vi "MainUI.vi"() -> ()   [LabVIEW 2017]
uses:
  QueueStates.ctl
  <vilib>/Instr/_visa.llb/VISA Configure Serial Port (Serial Instr).vi
panel:
  out "Phase Delta":dbl
  out "Gain":dbl
  out "Plot 1 PkPk":u16
  out "Plot 1 Min":u16
  out "Plot 1 Max":u16
  out "Plot 0 PkPk":u16
  in  "Sample Size":i32=1000
  out "Plot 0 Min":u16
  out "Plot 0 Max":u16
  out "Waveform Graph":u16[][](graph)
  out "String":string
  out "length":i32
  in  "Search Param":string="d"
  in  "STOP":bool
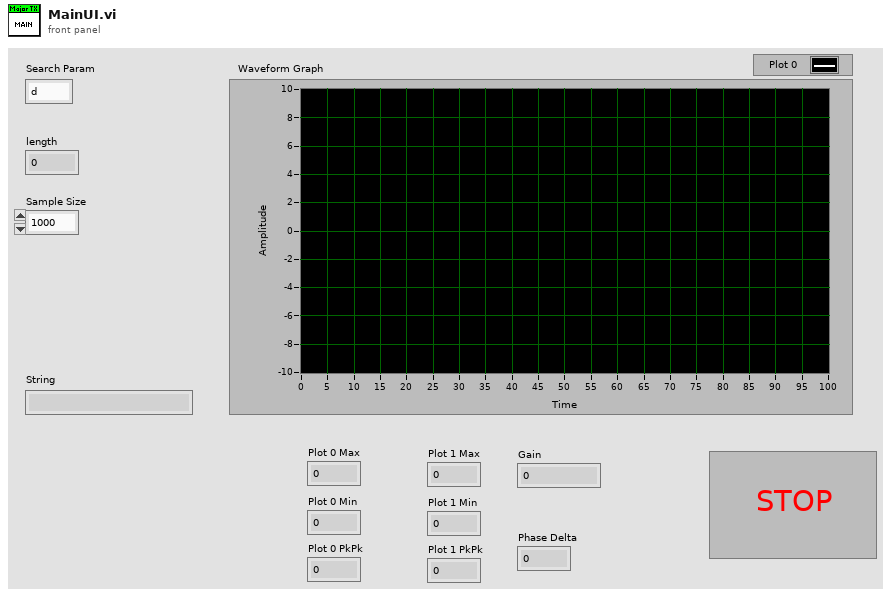
[diagram p1: front panel]
types:
  T1 = typedef "QueueStates.ctl" = enum16{"Init", "Exit", "Data", "CheckText", "Analyze"}
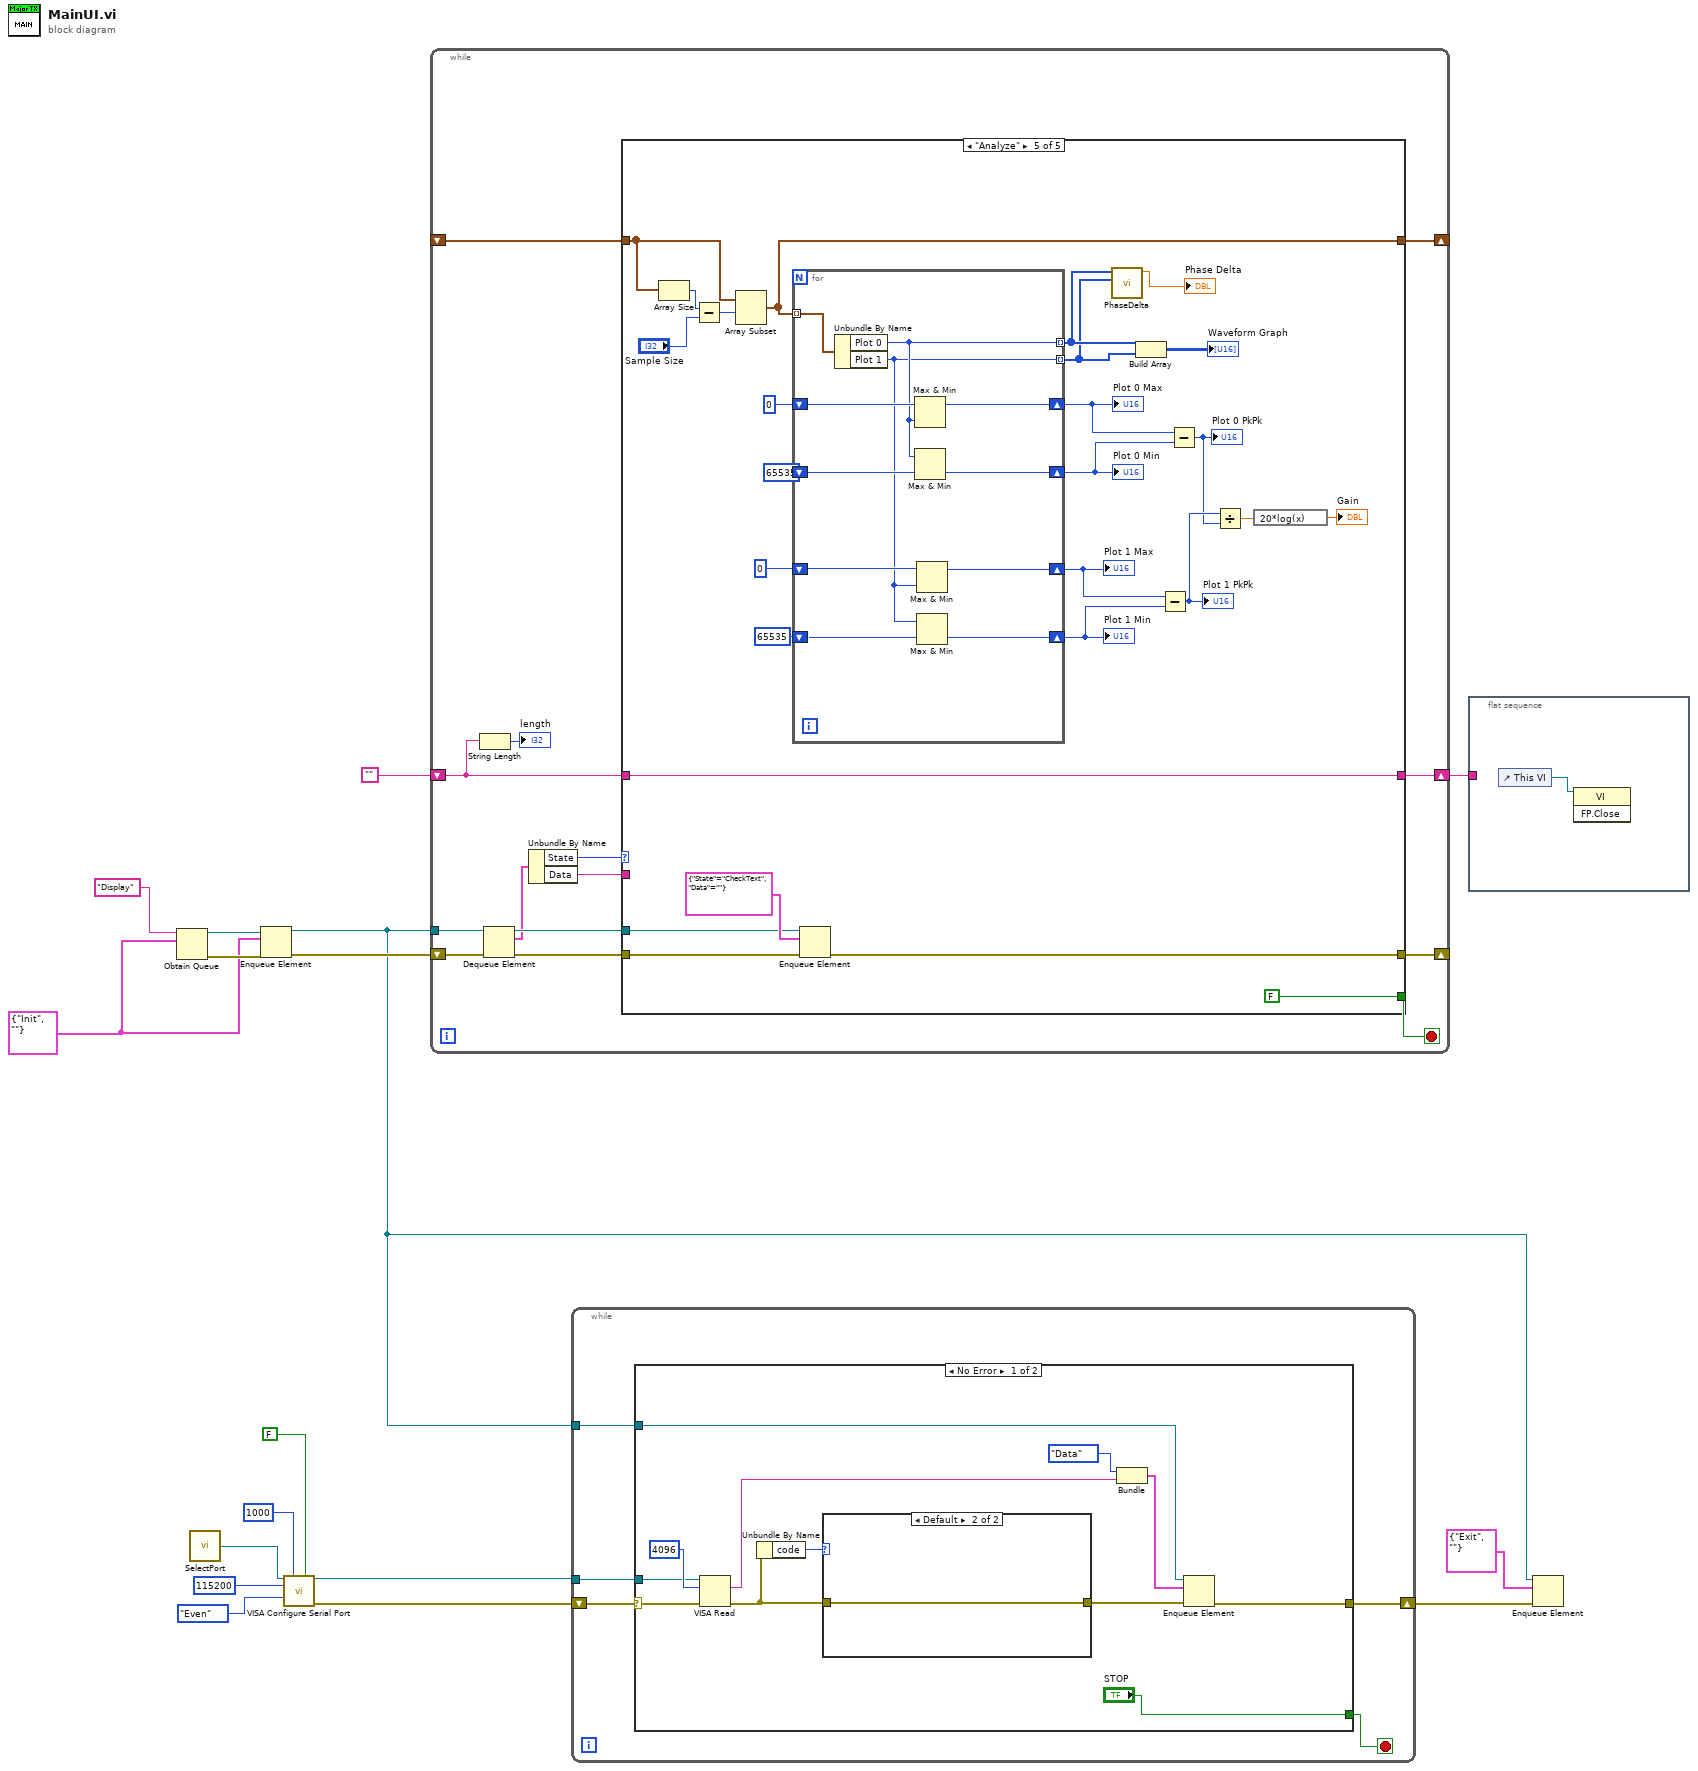
[diagram p0: block diagram]
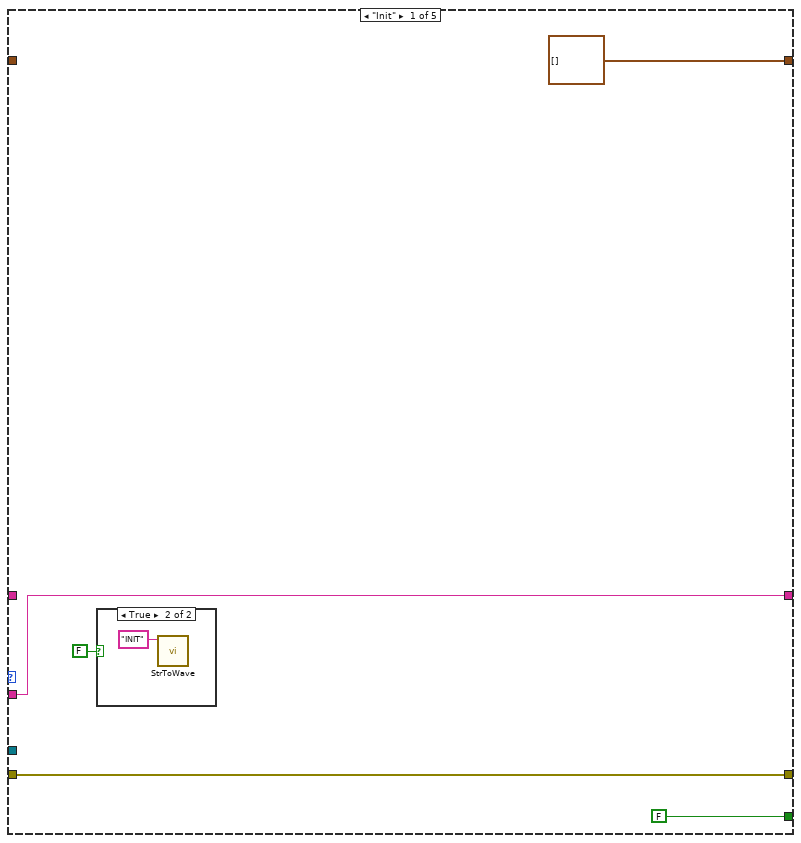
[diagram p2: hidden frame]
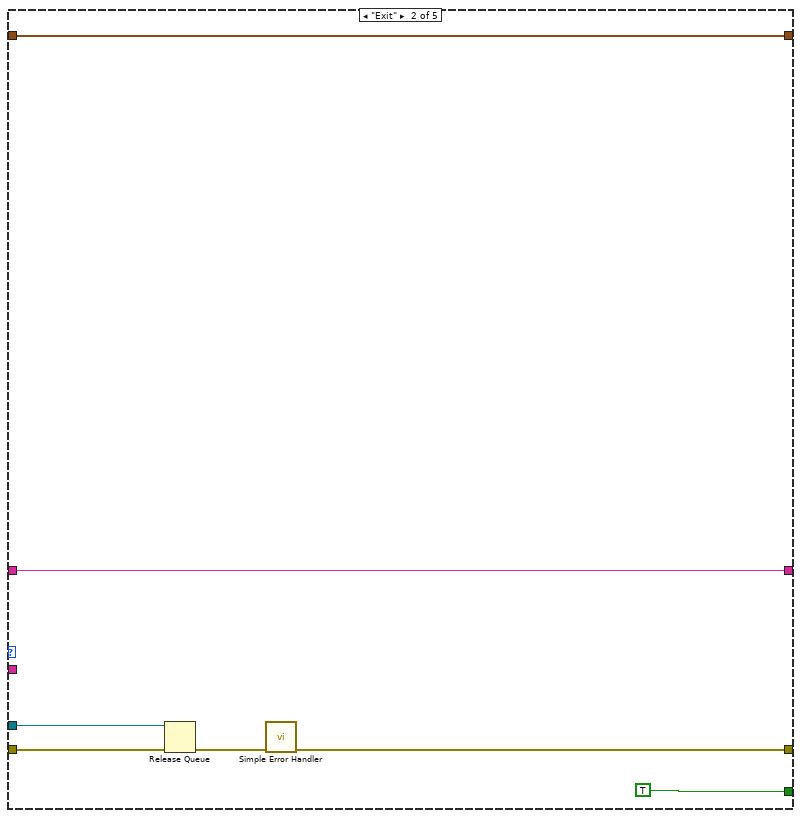
[diagram p4: hidden frame]
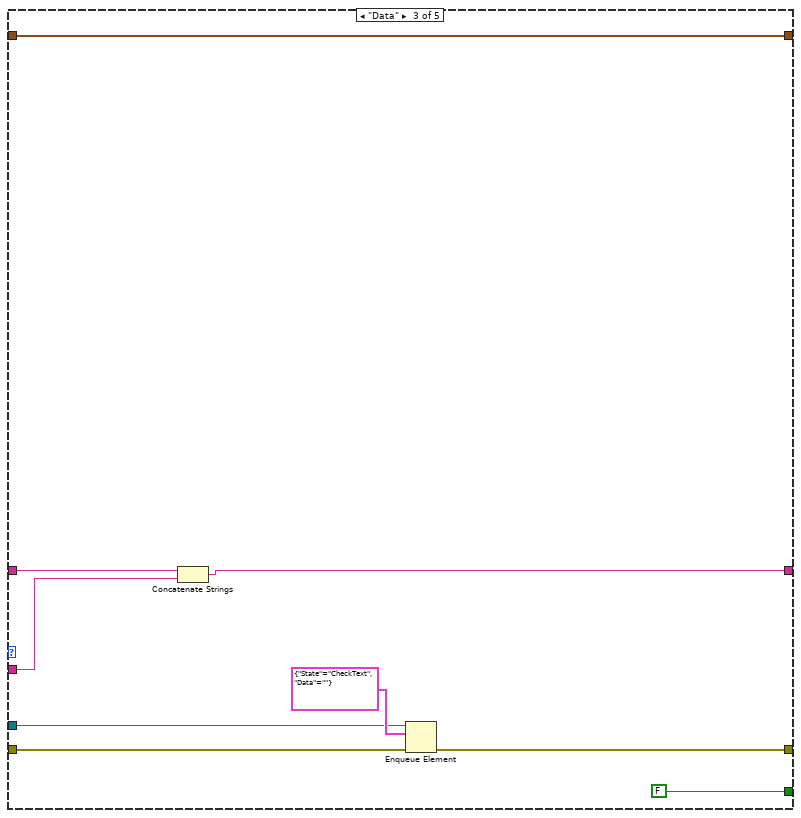
[diagram p5: hidden frame]
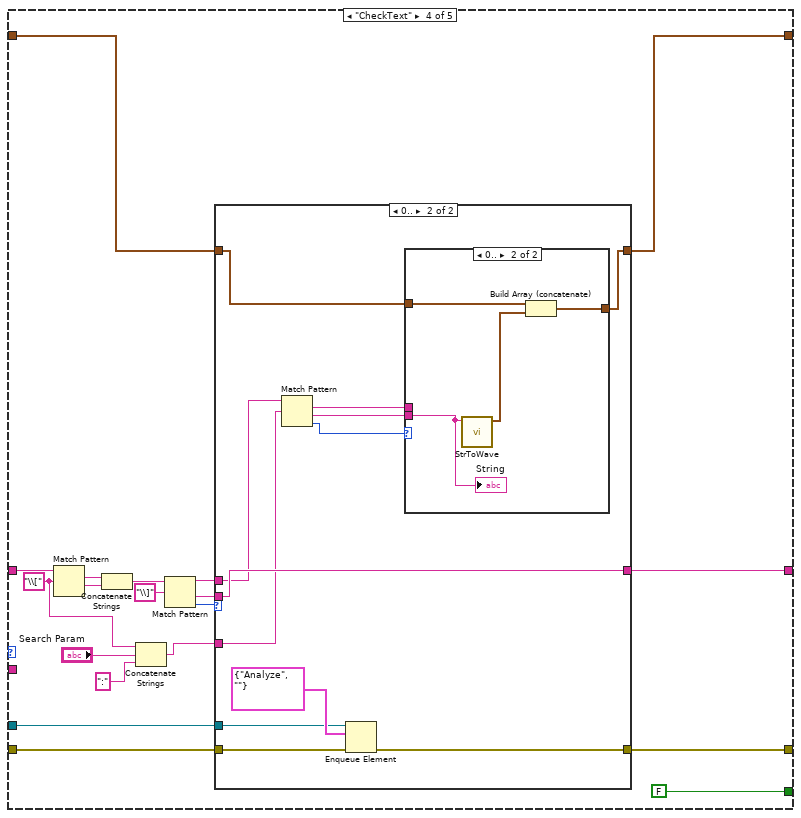
[diagram p6: hidden frame]
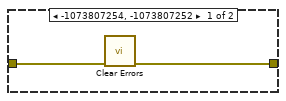
[diagram p9: hidden frame]
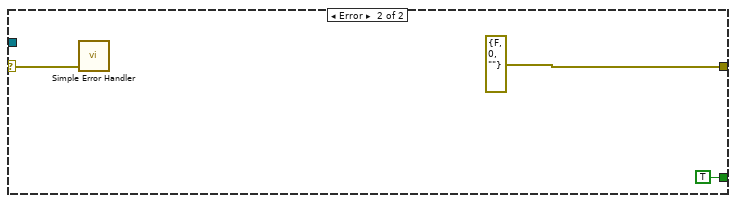
[diagram p10: hidden frame]
diagram:
  w7 = cluster{"State":T1, "Data":string} {"State"=enum."Init", "Data"=""}
  n1 = Obtain Queue(name (unnamed)="Display", element data type=w7) -> (queue out=w9:refnum<queue>, error out=w8:errorcluster)  [unwired: 3 in, 1 out]
  n2 = call "SelectPort.vi"() -> ("COM"=w17:refnum<visa-resource-name>)
  n3 = Enqueue Element(queue=w9, element=w7, error in (no error)=w8) -> (queue out=w5:refnum<queue>, error out=w6:errorcluster)  [unwired: 1 in, 1 out]
  n4 = call-poly "VISA Configure Serial Port"("VISA resource name"=w17, "timeout (10sec)"=u32 1000, "Enable Termination\nChar (T)"=FALSE ("Enable Termination\nChar (T)"), "baud rate (9600)"=u32 115200, "parity (0:none)"=enum16{"None", "Odd", "Even", "Mark", "Space"}."Even") -> ("VISA resource name out"=w12:refnum<visa-resource-name>, "error out"=w11:errorcluster)  [unwired: 9 in]
  n5 = while {
    tunnel: w5 -> [w21]
    shift-right: [w25] -> _
    shift-left: w6 -> [w31]
    shift-right: [w24] -> w1
    shift-left: "" -> [w23]
    shift-right: [w20] -> _
    shift-left: _ -> [w19]
    stop <- w18 stop-if-true
    n6 = String Length(string=w23) -> (length=→"length":i32)
    n7 = Dequeue Element(queue=w21, error in (no error)=w31) -> (queue out=w30:refnum<queue>, element=w29:cluster{"State":T1, "Data":string}, error out=w26:errorcluster)  [unwired: 1 in, 1 out]
    n8 = Unbundle By Name(w29) -> ("State"=w28:T1, "Data"=w27:string)
    n9 = case shown="\"Analyze\"" w28 {
      tunnel: w30 -> [_ w43 w46 w65 w117]
      tunnel: w27 -> [w36 _ w53 _ _]
      tunnel: w26 -> [w33 w42 w48 w64 w116]
      tunnel: [w33 w39 w47 w59 w115] -> w25
      tunnel: w23 -> [_ w41 w52 w72 w119]
      tunnel: [w36 w41 w51 w61 w119] -> w24
      tunnel: [FALSE TRUE FALSE FALSE FALSE] -> w18
      tunnel: [cluster{"Plot 0":u16, "Plot 1":u16}[] [] w38 w45 w55 w109] -> w20
      tunnel: w19 -> [_ w38 w45 w54 w111]
      frame "Init" {
        n10 = case shown="True" FALSE {
          frame False {
          }
          frame True {
            n11 = call "StrToWave.vi"("String"="INIT") -> ()  [unwired: 10 in, 1 out]
          }
        }
      }
      frame "Exit" {
        n12 = Release Queue(queue=w43, error in (no error)=w42) -> (error out=w40:errorcluster)  [unwired: 1 in, 2 out]
        n13 = call <vilib>:"Simple Error Handler.vi"("error in (no error)"=w40) -> ("error out"=w39:errorcluster)  [unwired: 4 in, 4 out]
      }
      frame "Data" {
        n14 = Concatenate Strings(w52, w53) -> (w51:string)
        n15 = Enqueue Element(queue=w46, element=cluster{"State":T1, "Data":string} {"State"=enum."CheckText", "Data"=""}, error in (no error)=w48) -> (error out=w47:errorcluster)  [unwired: 1 in, 2 out]
      }
      frame "CheckText" {
        w69 = "\\[" ("regular expression")
        n16 = Match Pattern(string=w72, regular expression=w69) -> (match substring=w71:string, after substring=w70:string)  [unwired: 1 in, 2 out]
        n17 = Concatenate Strings(w71, w70) -> (w67:string)
        n18 = Concatenate Strings(w69, "Search Param", ":" ("string")) -> (w57:string)
        n19 = Match Pattern(string=w67, regular expression="\\]") -> (before substring=w62:string, after substring=w60:string, offset past match=w63:i32)  [unwired: 1 in, 1 out]
        n20 = case shown="0.." w63 {
          tunnel: w65 -> [_ w86]
          tunnel: w64 -> [w74 w85]
          tunnel: w62 -> [w75 w81]
          tunnel: [w75 w83] -> w61
          tunnel: w60 -> [_ w83]
          tunnel: [w74 w84] -> w59
          tunnel: w57 -> [_ w82]
          tunnel: [w73 w76] -> w55
          tunnel: w54 -> [w73 w77]
          frame ..-1 {
          }
          frame 0.. {
            n21 = Match Pattern(string=w81, regular expression=w82) -> (match substring=w79:string, after substring=w78:string, offset past match=w80:i32)  [unwired: 1 in, 1 out]
            n22 = Enqueue Element(queue=w86, element=cluster{"State":T1, "Data":string} {"State"=enum."Analyze", "Data"=""}, error in (no error)=w85) -> (error out=w84:errorcluster)  [unwired: 1 in, 2 out]
            n23 = case shown="0.." w80 {
              tunnel: w79 -> [_ _]
              tunnel: w78 -> [_ w92]
              tunnel: w77 -> [w88 w91]
              tunnel: [w88 w89] -> w76
              frame ..-1 {
              }
              frame 0.. {
                n24 = call "StrToWave.vi"("String"=w92) -> ("Data"=w90:cluster{u16, u16})  [unwired: 10 in]
                n25 = Build Array (concatenate)(w91, w90) -> (w89:cluster{"Plot 0":u16, "Plot 1":u16}[])
                "String" <- w92
              }
            }
          }
        }
      }
      frame "Analyze" {
        n26 = Array Size(array=w111) -> (size(s)=w113:i32)
        n27 = Subtract(x=w113, y="Sample Size") -> (x-y=w110:i32)
        n28 = Array Subset(array=w111, index=w110) -> (w109:cluster{"Plot 0":u16, "Plot 1":u16}[])  [unwired: 1 in]
        n29 = for {
          tunnel: w109 -> [w130] mode=indexing
          tunnel: [w125] -> w95 mode=indexing
          tunnel: [w120] -> w94 mode=indexing
          shift-right: [w128] -> w105
          shift-left: u16 0 ("Plot 0 Max") -> [w129]
          shift-right: [w126] -> w104
          shift-left: u16 65535 ("Plot 0 Min") -> [w127]
          shift-right: [w123] -> w100
          shift-left: u16 0 ("Plot 1 Max") -> [w124]
          shift-right: [w122] -> w101
          shift-left: u16 65535 ("Plot 1 Min") -> [w121]
          n30 = Unbundle By Name(w130) -> ("Plot 0"=w125:u16, "Plot 1"=w120:u16)
          n31 = Max & Min(x=w129, y=w125) -> (max(x,y)=w128:u16)  [unwired: 1 out]
          n32 = Max & Min(x=w125, y=w127) -> (min(x,y)=w126:u16)  [unwired: 1 out]
          n33 = Max & Min(x=w124, y=w120) -> (max(x,y)=w123:u16)  [unwired: 1 out]
          n34 = Max & Min(x=w120, y=w121) -> (min(x,y)=w122:u16)  [unwired: 1 out]
        }
        "Plot 0 Max" <- w105
        "Plot 0 Min" <- w104
        "Plot 1 Max" <- w100
        "Plot 1 Min" <- w101
        n35 = Enqueue Element(queue=w117, element=cluster{"State":T1, "Data":string} {"State"=enum."CheckText", "Data"=""}, error in (no error)=w116) -> (error out=w115:errorcluster)  [unwired: 1 in, 2 out]
        n36 = call "PhaseDelta.vi"("Plot 1"=w94, "Plot 0"=w95) -> ("Phase Delta"=→"Phase Delta":dbl)  [unwired: 9 in]
        n37 = Build Array(w95, w94) -> (→"Waveform Graph":u16[][])
        n38 = Subtract(x=w100, y=w101) -> (x-y=w98:u16)
        "Plot 1 PkPk" <- w98
        n39 = Subtract(x=w105, y=w104) -> (x-y=w97:u16)
        "Plot 0 PkPk" <- w97
        n40 = Divide(x=w98, y=w97) -> (x/y=w99:dbl)
        n41 = expression code="20*log(x)"(w99) -> (→"Gain":dbl)
      }
    }
  }
  n42 = while {
    shift-right: [w134] -> w4
    shift-left: w11 -> [w135]
    tunnel: w12 -> [w132]
    tunnel: w5 -> [w131]
    stop <- w133 stop-if-true
    n43 = case shown="No Error" w135 {
      selector: w135 -> [w146 w151]
      tunnel: [w139 errorcluster {"status"=FALSE, "code"=0, "source"=""} ("error out")] -> w134
      tunnel: ["STOP" TRUE ("STOP")] -> w133
      tunnel: w132 -> [w144 _]
      tunnel: w131 -> [w143 _]
      frame No Error {
        n44 = VISA Read(VISA resource name=w144, byte count=u32 4096, error in (no error)=w146) -> (read buffer=w140:string, error out=w137:errorcluster)  [unwired: 2 out]
        n45 = Unbundle By Name(w137) -> ("code"=w138:i32)
        n46 = case shown="Default" w138 {
          tunnel: w137 -> [w149 w150]
          tunnel: [w148 w150] -> w136
          frame -1073807254, -1073807252 {
            n47 = call <vilib>:"Clear Errors.vi"("error in (no error)"=w149) -> ("error out"=w148:errorcluster)  [unwired: 5 in, 1 out]
          }
          frame Default {
          }
        }
        n48 = Bundle(QueueStates."Data", "read buffer"=w140) -> (w141:cluster{T1, "read buffer":string})  [unwired: 1 in]
        n49 = Enqueue Element(queue=w143, element=w141, error in (no error)=w136) -> (error out=w139:errorcluster)  [unwired: 1 in, 2 out]
      }
      frame Error {
        n50 = call <vilib>:"Simple Error Handler.vi"("error in (no error)"=w151) -> ()  [unwired: 4 in, 5 out]
      }
    }
  }
  n51 = flat-sequence {
    tunnel: w1 -> [_]
    frame #0 {
      n52 = control-ref of="This VI"() -> (w154:refnum<vi>)
      n53 = invoke class="VI" method="FP.Close"(reference=w154) -> ()  [unwired: 2 in, 3 out]
    }
  }
  n54 = Enqueue Element(queue=w5, element=cluster{"State":T1, "Data":string} {"State"=enum."Exit", "Data"=""}, error in (no error)=w4) -> ()  [unwired: 1 in, 3 out]
